vi "logging level t str.vi"(11 "level":u32(ring) items=["APDM_LL_ALL", "APDM_LL_DEBUG", "APDM_LL_INFO", "APDM_LL_WARNING", "APDM_LL_ERROR", "APDM_LL_NONE"]) -> (3 "function return":string)   [LabVIEW 2019, in "apdm.lvlib"]
doc: "APDM_EXPORT const char* apdm_logging_level_t_str(const apdm_logging_level_t level);"
uses:
  apdm.lvlib
  Lee Lab/CP FES Walking 2018/Code/Working/LabVIEW/apdm.dll
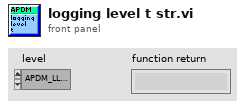
[diagram p1: front panel]
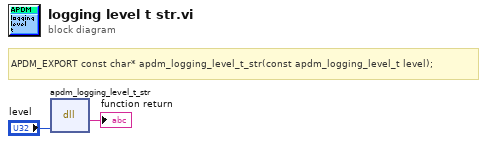
[diagram p0: block diagram]
diagram:
  # "APDM_EXPORT const char* apdm_logging_level_t_str(const apdm_logging_level_t level);"
  n1 = dll-call lib="C:/Users/jfalesi/Dropbox/Lee Lab/CP FES Walking 2018/Code/Working/LabVIEW/apdm.*" fn="apdm_logging_level_t_str"("level"="level") -> (→"function return":string)  [unwired: 4 in, 2 out]
